vi "Arduino Global.vi"() -> ()   [LabVIEW 2013]
uses:
  Arduino Config & resource typedef.ctl
panel:
  in  "Arduino VISA config & resource":T1[](array[typedef]) {"termination char (hex)" format="%02x"; "stop bits (10: 1 bit)" items=["1.0"=10, "1.5"=15, "2.0"=20]; "flow control" items=["None", "XON/XOFF", "RTS/CTS", "XON/XOFF & RTS/CTS", "DTR/DSR", "XON/XOFF & DTR/DSR"]}
  in  "Arduino VISA resource list":string[](array[string])
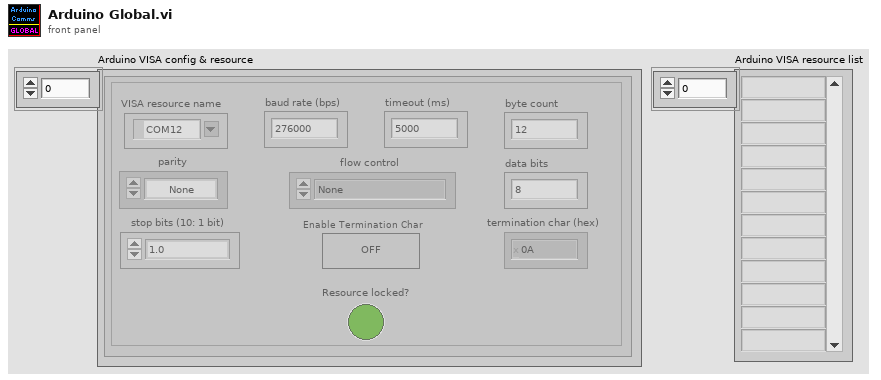
[diagram p1: front panel]
types:
  T1 = typedef "Arduino Config & resource typedef.ctl" = cluster{"VISA resource name":refnum<visa-resource-name>, "baud rate (bps)":u32, "timeout (ms)":u32, "data bits":u16, "parity":enum16{"None", "Odd", "Even", "Mark", "Space"}, "stop bits (10: 1 bit)":u16, "flow control":u16, "termination char (hex)":u8, "Enable Termination Char":bool, "byte count":u32, "Resource locked?":bool}
diagram:
